vi "GetPath.vi"(11 "GameName":string) -> (3 "appended path":path)   [LabVIEW 2019, in "RT_Game.lvlib" / "Highscore.lvclass"]
uses:
  Highscore.lvclass
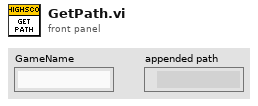
[diagram p1: front panel]
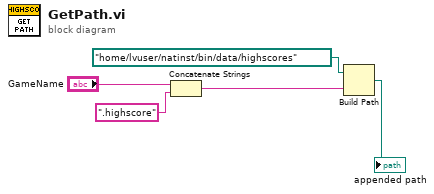
[diagram p0: block diagram]
diagram:
  n1 = Concatenate Strings("GameName", ".highscore" ("string")) -> (w5:string)
  n2 = Build Path(base path=path "/home/lvuser/natinst/bin/data/highscores" ("file path (use dialog)"), name or relative path=w5) -> (appended path=→"appended path":path)
